vi "Move.vi"(4 "Units (0: microsteps)":u16(ring) items=["microsteps", "microns", "millimeters", "inches"], 6 "Movement Type (0: relative)":u16(ring) items=["relative", "absolute"], 7 "Move Distance (0)":dbl, 8 "error in (no error)":errorcluster, 9 "Device and Axis":string, 10 "Microstep Size (0)":dbl, 11 "VISA resource name":refnum<visa-resource-name>) -> (0 "error out":errorcluster, 3 "VISA resource name out":refnum<visa-resource-name>)   [LabVIEW 2012, in "Zaber A Series.lvlib"]
doc: "Moves a device. You can optionally input the Device and Axis to move, and the other inputs specificy the type of movement (absolute or relative), the units of the data you'd like to send, and the distance data in those units. If no movement type or unit is input the default is relative movement in microsteps. Finally if you are using any other unit than microsteps you must input the Microstep Size for the model. \n\nNo responses are returned with this VI, but if you would like to wait until the movement is completed to continue, you can combine this VI with the Poll Until Idle VI. \n\nThis VI requires that the Initialize VI has been called with the same serial port. \n\nNote: See the Device Lookup control for the microstep size of your model, or check on the product specifications page for the product on www.zaber.com."
uses:
  <instrlib>/Zaber A Series/Zaber A Series.lvlib
  <instrlib>/Zaber A Series/Private/Basic Commands.ctl
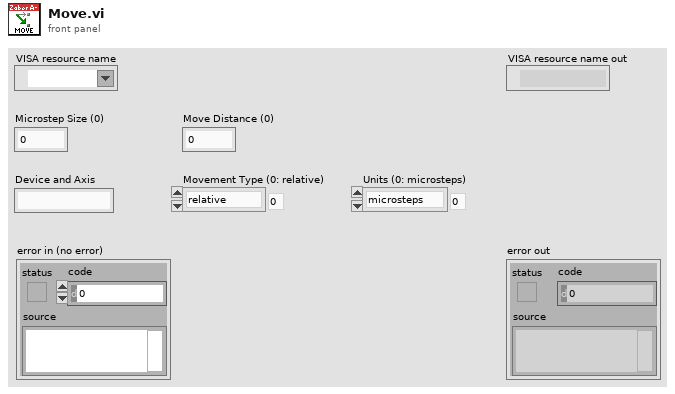
[diagram p1: front panel]
types:
  T1 = typedef "Zaber A Series.lvlib/Basic Commands.ctl" = string
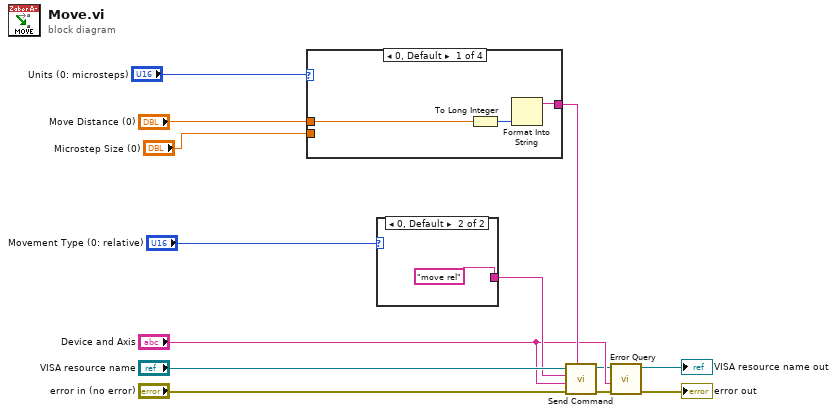
[diagram p0: block diagram]
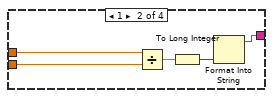
[diagram p2: hidden frame]
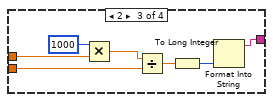
[diagram p3: hidden frame]
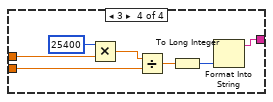
[diagram p4: hidden frame]
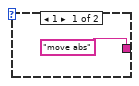
[diagram p5: hidden frame]
diagram:
  n1 = case shown="0, Default" "Units (0: microsteps)" {
    tunnel: "Move Distance (0)" -> [w16 w21 w25 w31]
    tunnel: [w14 w17 w26 w29] -> w7
    tunnel: "Microstep Size (0)" -> [_ w20 w22 w30]
    frame 0, Default {
      n2 = To Long Integer(number=w16) -> (32bit integer=w15:i32)
      n3 = Format Into String(w15) -> (resulting string=w14:string)  [unwired: 3 in, 1 out]
    }
    frame 1 {
      n4 = Divide(x=w21, y=w20) -> (x/y=w18:dbl)
      n5 = To Long Integer(number=w18) -> (32bit integer=w19:i32)
      n6 = Format Into String(w19) -> (resulting string=w17:string)  [unwired: 3 in, 1 out]
    }
    frame 2 {
      n7 = Multiply(x=1000, y=w25) -> (x*y=w23:dbl)
      n8 = Divide(x=w23, y=w22) -> (x/y=w28:dbl)
      n9 = To Long Integer(number=w28) -> (32bit integer=w27:i32)
      n10 = Format Into String(w27) -> (resulting string=w26:string)  [unwired: 3 in, 1 out]
    }
    frame 3 {
      n11 = Multiply(x=25400, y=w31) -> (x*y=w32:dbl)
      n12 = Divide(x=w32, y=w30) -> (x/y=w35:dbl)
      n13 = To Long Integer(number=w35) -> (32bit integer=w34:i32)
      n14 = Format Into String(w34) -> (resulting string=w29:string)  [unwired: 3 in, 1 out]
    }
  }
  n15 = case shown="0, Default" "Movement Type (0: relative)" {
    tunnel: [T1 "move abs" ("Basic Command List") T1 "move rel" ("Basic Command List")] -> w5
    frame 1 {
    }
    frame 0, Default {
    }
  }
  n16 = call <instrlib>:"Send Command.vi"("Data"=w7, "error in (no error)"="error in (no error)", "Device and Axis"="Device and Axis", "Command"=w5, "VISA resource name"="VISA resource name") -> ("error out"=w1:errorcluster, "VISA resource name out"=w2:refnum<visa-resource-name>)  [unwired: 2 in, 3 out]
  n17 = call <instrlib>:"Error Query.vi"("error in (no error)"=w1, "Device and Axis"="Device and Axis", "VISA resource name"=w2) -> ("error out"=→"error out":errorcluster, "VISA resource name out"=→"VISA resource name out":refnum<visa-resource-name>)  [unwired: 5 in, 2 out]
